vi "WLAN - niVST - RFSA - Gain and Trigger Settings_5663.vi"(0 "instrument handle":refnum<k15>, 7 "External Attenuation (dB)":dbl, 11 "error in":errorcluster) -> (4 "instrument handle":refnum<k15>, 15 "error out":errorcluster)   [LabVIEW 2011]
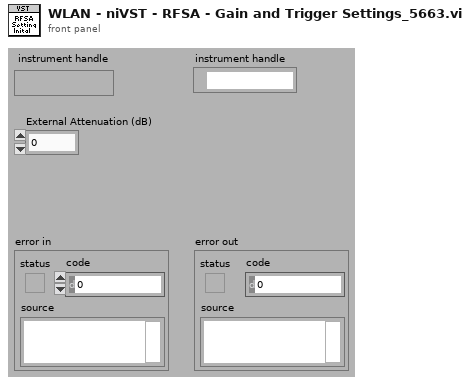
[diagram p1: front panel]
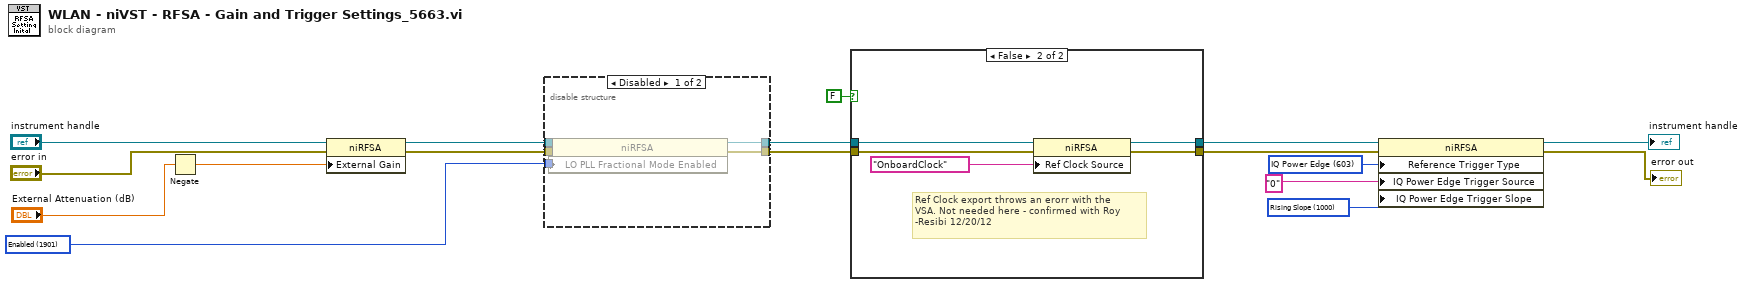
[diagram p0: block diagram]
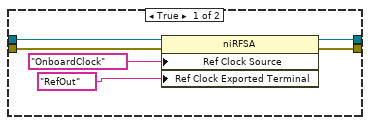
[diagram p2: hidden frame]
diagram:
  w11 = 1000 items=["Rising Slope"=1000, "Falling Slope"=1001] ("Triggers:Ref:IQ Power Edge:Slope")
  w13 = 603 items=["None"=600, "Digital Edge"=601, "IQ Power Edge"=603, "Software"=604, "IQ Analog Edge"=605] ("Triggers:Ref:Type")
  w2 = 1901 items=["Disabled"=1900, "Enabled"=1901] ("RF-RIO:Signal Path:LO PLL Fractional Mode Enabled")
  n1 = Negate(x="External Attenuation (dB)") -> (-x=w14:dbl)
  n2 = property on="Property Node" class="niRFSA"(reference="instrument handle", error in="error in", "External Gain"=w14) -> (reference out=w6:refnum<k15>, error out=w3:errorcluster)
  n3 = disable-structure shown="Disabled" {
    disable-tunnel: w6 -> [w22 w23]
    disable-tunnel: [w21 w23] -> w5
    disable-tunnel: [w20 w24] -> w4
    disable-tunnel: w3 -> [w19 w24]
    disable-tunnel: w2 -> [w18 _]
    frame Disabled {
      n4 = property on="Property Node" class="niRFSA"(reference=w22, error in=w19, "LO PLL Fractional Mode Enabled"=w18) -> (reference out=w21:refnum<k15>, error out=w20:errorcluster)
    }
    frame Enabled {
    }
  }
  n5 = case shown="False" FALSE {
    tunnel: [w29 w34] -> w10
    tunnel: [w28 w33] -> w9
    tunnel: w5 -> [w27 w32]
    tunnel: w4 -> [w26 w31]
    frame True {
      n6 = property class="niRFSA"(reference=w27, error in=w26, "Ref Clock Source"="OnboardClock" ("Clocking:Ref Clock Source"), "Ref Clock Exported Terminal"="RefOut" ("Clocking:Ref Clock Exported Terminal")) -> (reference out=w29:refnum<k15>, error out=w28:errorcluster)
    }
    frame False {
      # "Ref Clock export throws an erorr with the \nVSA. Not needed here - confirmed with Roy\n-Resibi 12/20/12"
      n7 = property class="niRFSA"(reference=w32, error in=w31, "Ref Clock Source"="OnboardClock" ("Clocking:Ref Clock Source")) -> (reference out=w34:refnum<k15>, error out=w33:errorcluster)
    }
  }
  n8 = property class="niRFSA"(reference=w10, error in=w9, "Reference Trigger Type"=w13, "IQ Power Edge Trigger Source"="0" ("source"), "IQ Power Edge Trigger Slope"=w11) -> (reference out=→"instrument handle":refnum<k15>, error out=→"error out":errorcluster)
